vi "CRYFlatten Recall.vi"(11 "Recall":T1={"Name"="Test for Signal [L]", "filepath"="Test for Signal [L]", "all or last"=0, "File Path Mode"=0, "Curve Names"=[], "format string"={"dB Format String out"="", "Lin Format String out"=""}, "Template"=[], "Axis"=0, "*.imp Path"=path "", "Filepath option"=0, "ML Value"=0.0, "user defined"="Test for Signal [L]", "Curves Selected?"=[], "Help"="", "Tab Value"=enum."Setting", "Selector"=0, "Use Default"=FALSE} {"Selector" items=["Space", "Underscores", "None"]; "Axis" scale=0.0..2.0; "Template" format="%#.0f"}) -> (3 "Recall flattened":string)   [LabVIEW 2013]
uses:
  Typedef Control/CRYRecall Cluster.ctl
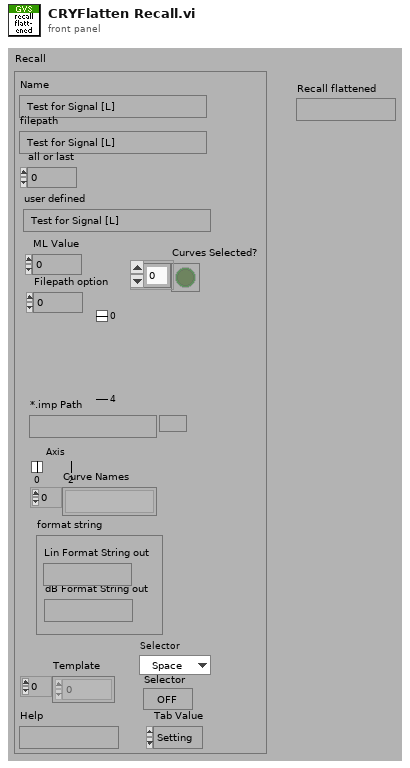
[diagram p1: front panel]
types:
  T1 = typedef "CRYRecall Cluster.ctl" = cluster{"Name":string, "filepath":string, "all or last":i32, "File Path Mode":u16, "Curve Names":string[], "format string":cluster{"dB Format String out":string, "Lin Format String out":string}, "Template":u16[], "Axis":u16, "*.imp Path":path, "Filepath option":i16, "ML Value":dbl, "user defined":string, "Curves Selected?":bool[], "Help":string, "Tab Value":enum32{"Setting", "Help"}, "Selector":i32, "Use Default":bool}
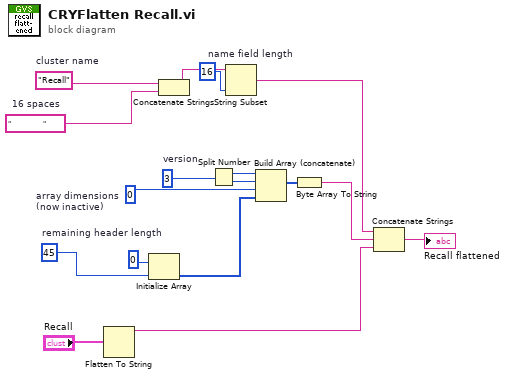
[diagram p0: block diagram]
diagram:
  w3 = u8 0  # array dimensions (now inactive)
  w6 = 16  # name field length
  w7 = "                "  # 16 spaces
  w8 = "Recall"  # cluster name
  w13 = 45  # remaining header length
  w17 = u16 3  # version
  n1 = Flatten To String(anything="Recall") -> (data string=w2:string)  [unwired: 1 in, 4 out]
  n2 = Initialize Array(u8 0, w13) -> (w9:u8[])
  n3 = Concatenate Strings(w8, w7) -> (w5:string)
  n4 = Split Number(x=w17) -> (hi(x)=w16:u8, lo(x)=w15:u8)
  n5 = String Subset(string=w5, length (rest)=w6) -> (substring=w4:string)  [unwired: 1 out]
  n6 = Build Array (concatenate)(w16, w15, w3, w9) -> (w12:u8[])
  n7 = Byte Array To String(unsigned byte array=w12) -> (string=w10:string)
  n8 = Concatenate Strings(w4, w10, w2) -> (→"Recall flattened":string)
